vi "Parse Trip.vi"(10 "Trip":enum16{"Trip A", "Trip B", "Trip C", "Trip D"}(ring), 11 "Buffer in":string) -> (1 "Trip Pressure":dbl, 2 "Trip Association":string, 3 "Buffer out":string)   [LabVIEW 2019, in "PGC2D.lvlib"]
uses:
  PGC2D.lvlib
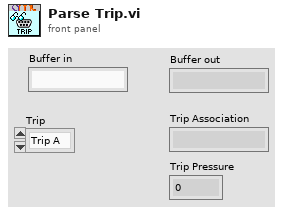
[diagram p1: front panel]
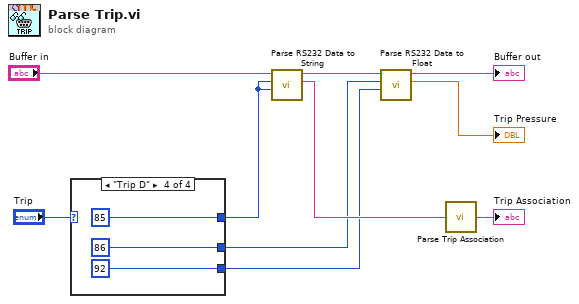
[diagram p0: block diagram]
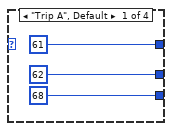
[diagram p2: hidden frame]
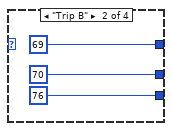
[diagram p3: hidden frame]
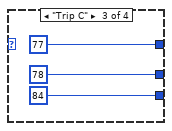
[diagram p4: hidden frame]
diagram:
  n1 = case shown="\"Trip D\"" "Trip" {
    tunnel: [61 ("AML end byte") 69 ("AML end byte") 77 ("AML end byte") 85 ("AML end byte")] -> w4
    tunnel: [68 ("AML end byte") 76 ("AML end byte") 84 ("AML end byte") 92 ("AML end byte")] -> w2
    tunnel: [62 ("AML start byte") 70 ("AML start byte") 78 ("AML start byte") 86 ("AML start byte")] -> w1
    frame "Trip A", Default {
    }
    frame "Trip B" {
    }
    frame "Trip C" {
    }
    frame "Trip D" {
    }
  }
  n2 = call "Parse RS232 Data to String.vi"("AML end byte"=w4, "AML start byte"=w4, "bytes in"="Buffer in") -> ("string data"=w8:string, "bytes out"=w9:string)  [unwired: 7 in]
  n3 = call "Parse RS232 Data to Float.vi"("AML end byte"=w2, "AML start byte"=w1, "bytes in"=w9) -> ("DBL data"=→"Trip Pressure":dbl, "bytes out"=→"Buffer out":string)  [unwired: 7 in]
  n4 = call "Parse Trip Association.vi"("Buffer in"=w8) -> ("trip"=→"Trip Association":string)
